vi "GD_Insert_data.vi"(8 "error in (no error)":errorcluster, 10 "carrier":i16, 11 "DBlink":string="Driver={ODBC Driver 17 for SQL Server};Server=localhost\\SQLEXPRESS;Database=ZDX201;UID=labview;PWD=Dsa@54137926") -> (0 "error out":errorcluster={"status"=TRUE, "code"=-2147217900, "source"="NI_Database_API.lvlib:Cmd Execute.vi->NI_Database_API.lvlib:DB Tools Insert Data.vi->GD_Insert_data.vi<ERR>ADO Error: 0x80040E14\r\nException occured in Microsoft OLE DB Provider for ODBC Drivers: [Microsoft][ODBC Driver 17 for SQL Server][SQL Server]無法插入 NULL 值到資料行 'update_time'，資料表 'ZDX201.dbo.glue_data'; 資料行不得有 Null。INSERT 失敗。 in NI_Database_API.lvlib:Rec Create - Command.vi->NI_Database_API.lvlib:Cmd Execute.vi->NI_Database_API.lvlib:DB Tools Insert Data.vi->GD_Insert_data.vi"}, 2 "id":string)   [LabVIEW 2019]
uses:
  <vilib>/addons/database/Connection.llb/DB Tools Open Connec (String).vi
  <vilib>/addons/database/Connection.llb/Conn Execute.vi
  <vilib>/addons/database/Recordset.llb/Rec Fetch Recordset Data (R).vi
  <vilib>/addons/database/Recordset.llb/Rec Destroy - Connection.vi
  <vilib>/addons/database/_DB Variant To Data/Database Variant To Data.xnode
  <vilib>/addons/database/NI_Database_API.lvlib
panel:
  in  "columns":string[](array[string])=["time_supply", "glue_workspace_id", "update_time", "[carrier_num]"]
  in  "Insert value":T1={"Time_supply"=timestamp(3733895123.4509425 s since 1904-01-01), "[glue_workspace_id]"=1, "update_time"=timestamp(3733895123.4509425 s since 1904-01-01), "carrier_num"=1} {"update_time" format="%<%.0X %x>T"; "Time_supply" format="%<%.0X %x>T"}
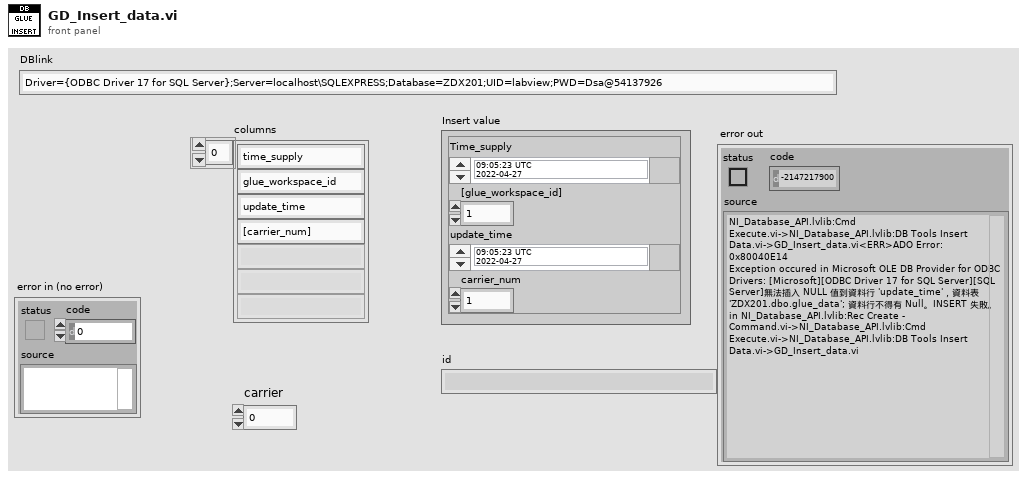
[diagram p1: front panel]
types:
  T1 = cluster{"Time_supply":timestamp, "[glue_workspace_id]":i16, "update_time":timestamp, "carrier_num":i16}
  T2 = typedef "NI_Database_API.lvlib/Conn ObjectReference.ctl" = refnum<k1>
  T3 = typedef "NI_Database_API.lvlib/Rec ObjectReference.ctl" = refnum<k1>
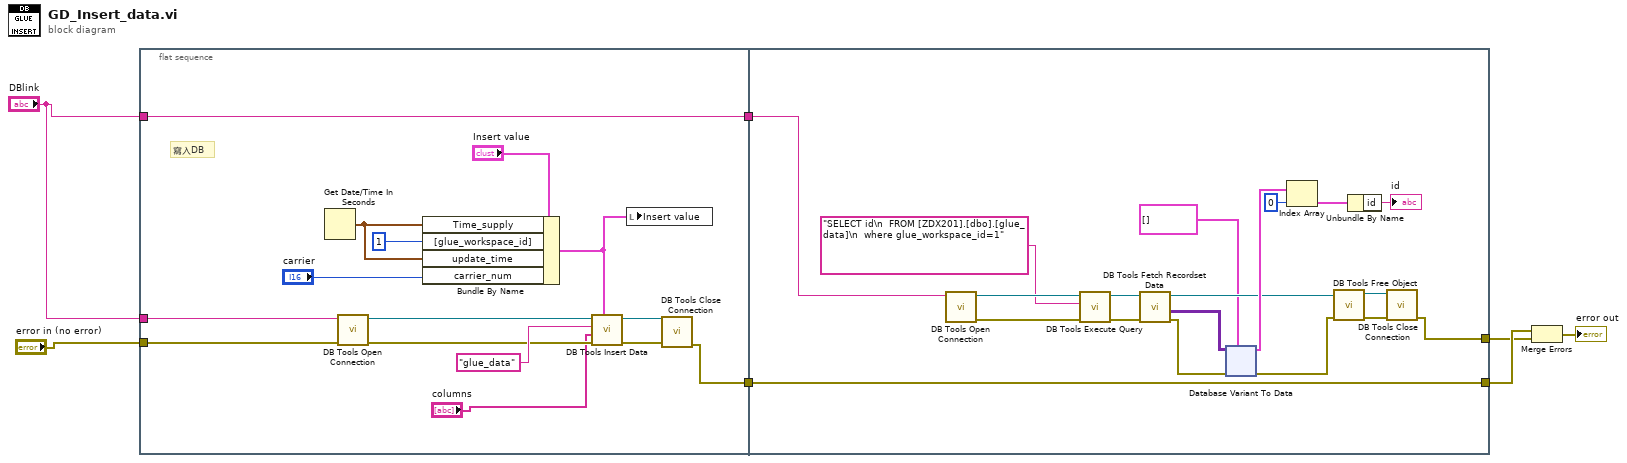
[diagram p0: block diagram]
diagram:
  n1 = flat-sequence {
    tunnel: "error in (no error)" -> [w13]
    tunnel: "DBlink" -> [w11]
    tunnel: [w10] -> w6
    tunnel: "DBlink" -> [w10]
    tunnel: [w9] -> w3
    tunnel: w6 -> [w25]
    tunnel: [w24] -> w4
    tunnel: w3 -> [w24]
    tunnel: [w23] -> w2
    frame #0 {
      # "寫入DB"
      n2 = Get Date/Time In Seconds() -> (seconds since 1Jan1904=w12:timestamp)
      n3 = call-poly <vilib>:"DB Tools Open Connection.vi"("error in (no error)"=w13, "connection information"=w11) -> ("error out"=w19:errorcluster, "connection reference"=w18:T2)  [unwired: 6 in]
      n4 = Bundle By Name(cluster="Insert value", "Time_supply"=w12, "[glue_workspace_id]"=i16 1 ("workspace"), "update_time"=w12, "carrier_num"="carrier") -> (w16:T1)
      n5 = call <vilib>:"DB Tools Insert Data.vi"("data"=w16, "error in (no error)"=w19, "columns"="columns", "table"="glue_data", "connection reference"=w18) -> ("error out"=w21:errorcluster, "connection reference out"=w22:T2)  [unwired: 5 in]
      n6 = local write "Insert value"(w16) -> ()
      n7 = call <vilib>:"DB Tools Close Connection.vi"("error in (no error)"=w21, "connection reference"=w22) -> ("error out"=w9:errorcluster)  [unwired: 5 in]
    }
    frame #1 {
      n8 = call-poly <vilib>:"DB Tools Open Connection.vi"("connection information"=w25) -> ("error out"=w37:errorcluster, "connection reference"=w36:T2)  [unwired: 7 in]
      n9 = call-poly <vilib>:"DB Tools Execute Query.vi"("error in (no error)"=w37, "SQL query"="SELECT id\n  FROM [ZDX201].[dbo].[glue_data]\n  where glue_workspace_id=1", "connection reference"=w36) -> ("error out"=w34:errorcluster, "recordset reference"=w35:T3)  [unwired: 5 in]
      n10 = call-poly <vilib>:"DB Tools Fetch Recordset Data.vi"("error in (no error)"=w34, "recordset reference"=w35) -> ("error out"=w29:errorcluster, "recordset data"=w39:variant[][], "recordset reference out"=w30:T3)  [unwired: 3 in]
      n11 = xnode "Database Variant To Data"("database variant"=w39, "error in (no error)"=w29, "type"=cluster{"id":string}[] [] ("Workplace: assemble")) -> ("data"=w38:cluster{"id":string}[], "error out"=w31:errorcluster)
      n12 = Index Array(array=w38, index=0) -> (element=w40:cluster{"id":string})
      n13 = call-poly <vilib>:"DB Tools Free Object.vi"("error in (no error)"=w31, "recordset reference"=w30) -> ("error out"=w32:errorcluster, "connection reference"=w33:T2)  [unwired: 8 in]
      n14 = Unbundle By Name(w40) -> ("id"=→"id":string)
      n15 = call <vilib>:"DB Tools Close Connection.vi"("error in (no error)"=w32, "connection reference"=w33) -> ("error out"=w23:errorcluster)  [unwired: 5 in]
    }
  }
  n16 = Merge Errors(w4, w2) -> (→"error out":errorcluster)
